vi "test_libssh2_userauth_banner.vi"() -> ()   [LabVIEW 2017, in "integration_tests.lvlib"]
uses:
  integration_tests.lvlib
  libssh2/libssh2_session_handshake_tcp.vi
  libssh2/libssh2_init_default.vi
  libssh2/libssh2_session_init_ex.vi
  <vilib>/Utility/tcp.llb/TCP Get Raw Net Object.vi
  libssh2/libssh2_session_handshake_socket.vi
  libssh2/libssh2.lvlib
  support/support.lvlib
  <vilib>/PNR/Transparent Assertions/Transparent Assertions/Transparent Assertions.lvlib
panel:
  out "error out":errorcluster
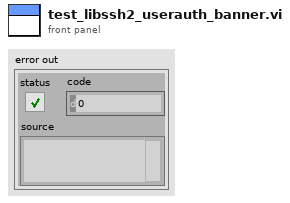
[diagram p1: front panel]
types:
  T1 = typedef "libssh2.lvlib/Session Refnum.ctl" = refnum<k1>
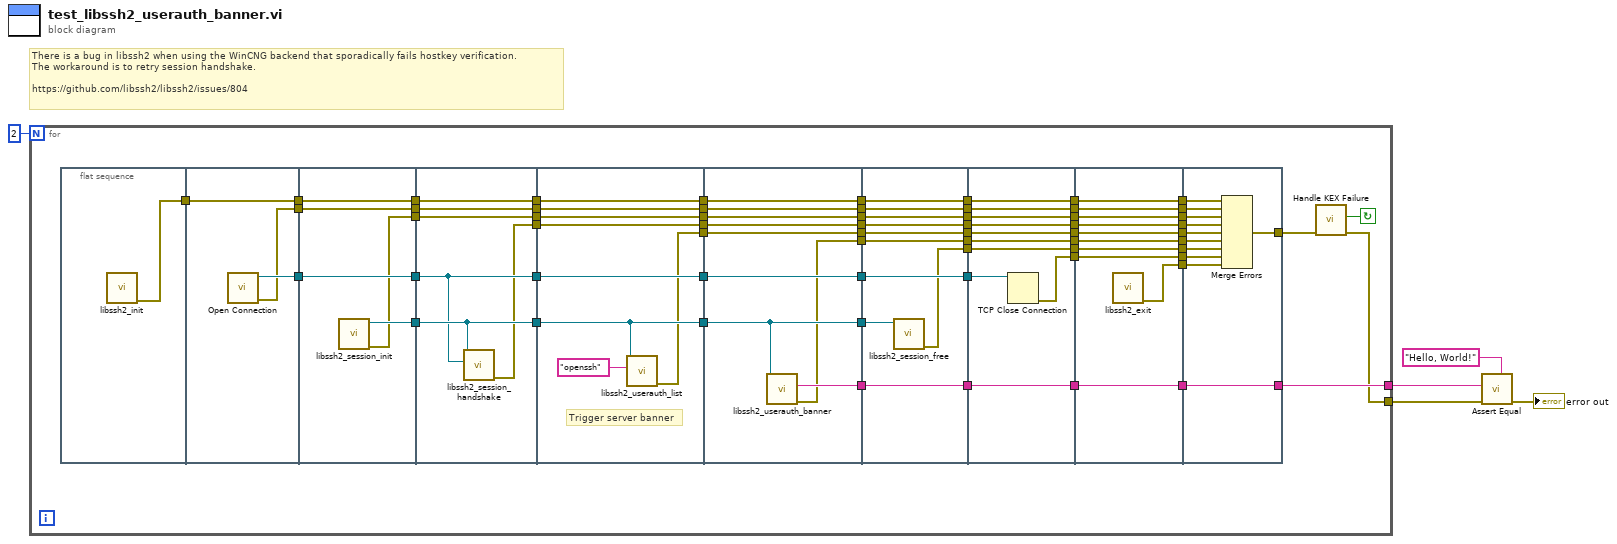
[diagram p0: block diagram]
diagram:
  # "There is a bug in libssh2 when using the WinCNG backend that sporadically fails hostkey verification.\nThe workaround is to retry session handshake.\n\nhttps://github.com/libssh2/libssh2/issues/804"
  n1 = for {
    N: 2 -> [_]
    tunnel: [w9] -> w3
    tunnel: [w6] -> w2
    stop <- w7 continue-if-true
    n2 = flat-sequence {
      tunnel: [w69] -> w68
      tunnel: [w72] -> w67
      tunnel: w68 -> [w71]
      tunnel: [w71] -> w66
      tunnel: [w70] -> w65
      tunnel: w67 -> [w77]
      tunnel: [w77] -> w64
      tunnel: w66 -> [w76]
      tunnel: [w76] -> w63
      tunnel: w65 -> [w75]
      tunnel: [w75] -> w62
      tunnel: [w74] -> w61
      tunnel: [w73] -> w60
      tunnel: w64 -> [w79]
      tunnel: [w79] -> w59
      tunnel: w63 -> [w83]
      tunnel: [w83] -> w58
      tunnel: w62 -> [w82]
      tunnel: [w82] -> w57
      tunnel: [w81] -> w56
      tunnel: w61 -> [w81]
      tunnel: w60 -> [w80]
      tunnel: [w80] -> w55
      tunnel: [w78] -> w54
      tunnel: w59 -> [w91]
      tunnel: [w91] -> w53
      tunnel: w58 -> [w90]
      tunnel: [w90] -> w52
      tunnel: w57 -> [w89]
      tunnel: [w89] -> w51
      tunnel: w56 -> [w86]
      tunnel: w55 -> [w88]
      tunnel: [w88] -> w50
      tunnel: w54 -> [w87]
      tunnel: [w87] -> w49
      tunnel: [w86] -> w48
      tunnel: [w84] -> w47
      tunnel: w53 -> [w100]
      tunnel: [w100] -> w46
      tunnel: w52 -> [w99]
      tunnel: [w99] -> w45
      tunnel: w51 -> [w98]
      tunnel: [w98] -> w44
      tunnel: w50 -> [w97]
      tunnel: [w97] -> w43
      tunnel: w49 -> [w96]
      tunnel: [w96] -> w42
      tunnel: w48 -> [w95]
      tunnel: [w95] -> w41
      tunnel: [w94] -> w40
      tunnel: w47 -> [w93]
      tunnel: [w93] -> w39
      tunnel: [w92] -> w38
      tunnel: w46 -> [w110]
      tunnel: [w110] -> w37
      tunnel: w45 -> [w109]
      tunnel: [w109] -> w36
      tunnel: w44 -> [w108]
      tunnel: [w108] -> w35
      tunnel: w43 -> [w107]
      tunnel: [w107] -> w34
      tunnel: w42 -> [w106]
      tunnel: [w106] -> w33
      tunnel: [w105] -> w32
      tunnel: [w103] -> w31
      tunnel: w41 -> [w104]
      tunnel: w40 -> [w103]
      tunnel: w39 -> [w102]
      tunnel: [w102] -> w30
      tunnel: w38 -> [w101]
      tunnel: [w101] -> w29
      tunnel: w37 -> [w120]
      tunnel: w36 -> [w119]
      tunnel: [w119] -> w28
      tunnel: w35 -> [w118]
      tunnel: [w118] -> w27
      tunnel: [w117] -> w26
      tunnel: w34 -> [w116]
      tunnel: [w116] -> w25
      tunnel: w33 -> [w115]
      tunnel: [w115] -> w24
      tunnel: [w114] -> w23
      tunnel: w32 -> [w114]
      tunnel: [w113] -> w22
      tunnel: w31 -> [w113]
      tunnel: w30 -> [w112]
      tunnel: [w112] -> w21
      tunnel: w29 -> [w111]
      tunnel: [w111] -> w20
      tunnel: w28 -> [w130]
      tunnel: [w130] -> w19
      tunnel: w27 -> [w129]
      tunnel: [w129] -> w18
      tunnel: w26 -> [w128]
      tunnel: [w128] -> w17
      tunnel: [w127] -> w16
      tunnel: w25 -> [w126]
      tunnel: [w126] -> w15
      tunnel: w24 -> [w125]
      tunnel: [w125] -> w14
      tunnel: [w124] -> w13
      tunnel: w23 -> [w124]
      tunnel: [w123] -> w12
      tunnel: w22 -> [w123]
      tunnel: w21 -> [w122]
      tunnel: [w122] -> w11
      tunnel: w20 -> [w121]
      tunnel: [w121] -> w10
      tunnel: w19 -> [w141]
      tunnel: w18 -> [w140]
      tunnel: w17 -> [w139]
      tunnel: w16 -> [w138]
      tunnel: w15 -> [w137]
      tunnel: w14 -> [w136]
      tunnel: w13 -> [w135]
      tunnel: w12 -> [w132]
      tunnel: w11 -> [w134]
      tunnel: w10 -> [w133]
      tunnel: [w132] -> w9
      tunnel: [w131] -> w8
      frame #0 {
        n3 = call-poly "libssh2_init.vi"() -> ("error out"=w69:errorcluster)  [unwired: 11 in]
      }
      frame #1 {
        n4 = call "Open Connection.vi"() -> ("error out"=w70:errorcluster, "connection ID"=w72:refnum<k5>)  [unwired: 10 in]
      }
      frame #2 {
        n5 = call "libssh2_session_init.vi"() -> ("error out"=w73:errorcluster, "session"=w74:T1)  [unwired: 10 in]
      }
      frame #3 {
        n6 = call-poly "libssh2_session_handshake.vi"("tcp connection"=w79, "session"=w81) -> ("error out"=w78:errorcluster)  [unwired: 9 in]
      }
      frame #4 {
        # "Trigger server banner"
        n7 = call "libssh2_userauth_list.vi"("username"="openssh", "session"=w86) -> ("error out"=w84:errorcluster)  [unwired: 8 in, 1 out]
      }
      frame #5 {
        n8 = call "libssh2_userauth_banner.vi"("session"=w95) -> ("error out"=w92:errorcluster, "banner"=w94:string)  [unwired: 9 in]
      }
      frame #6 {
        n9 = call "libssh2_session_free.vi"("session"=w104) -> ("error out"=w105:errorcluster)  [unwired: 10 in]
      }
      frame #7 {
        n10 = TCP Close Connection(connection ID=w120) -> (error out=w117:errorcluster)  [unwired: 2 in, 1 out]
      }
      frame #8 {
        n11 = call "libssh2_exit.vi"() -> ("error out"=w127:errorcluster)  [unwired: 11 in]
      }
      frame #9 {
        n12 = Merge Errors(w141, w140, w137, w136, w134, w133, w135, w139, w138) -> (w131:errorcluster)
      }
    }
    n13 = call "Handle KEX Failure.vi"("error in (no error)"=w8) -> ("error out"=w6:errorcluster, "KEX Failure"=w7:bool)  [unwired: 9 in]
  }
  n14 = call <vilib>:"Assert Equal.vi"("Expected"="Hello, World!" ("banner"), "error in (no error)"=w2, "Actual"=w3) -> ("error out"=→"error out":errorcluster)  [unwired: 8 in]
